vi "Main.vi"() -> ()   [LabVIEW 2015, in "Stock.lvlib"]
doc: "This template is based off of the Queued Message Handler design pattern and the Queued Message Handler project template that ships with LabVIEW.\n\nThe main difference is that the queue is private to this module and communication between modules is performed via Broadcast and Request events.\n\nRequest events are wrapped in public API methods and are handled in the Event Handling Loop (EHL) of this VI. Any module can register for Broadcast events sent by this module. The EHL generates messages based on user interface actions.\n\nThe Message Handling Loop (MHL) processes messages generated by the EHL, or by other messages. The messages are string values, so new messages can be added easily to the Message Cases case structure in the MHL. Each message cluster can also provide an optional value for Message Data, which is a variant that can be converted to whatever message-specific data is required.\n_____\nBased on Delacor QMH Project Template 4.2.1.64."
uses:
  Stock.lvlib
  <vilib>/Delacor/Delacor QMH/Libraries/Module Admin_class/Delacor_lib_QMH_Module Admin.lvclass
  Module Data--cluster.ctl
  Products.ctl
  <vilib>/Delacor/Delacor QMH/Libraries/Message Queue_class/Delacor_lib_QMH_Message Queue.lvclass/Delacor_lib_QMH_Message Queue.ctl
  Stop Argument--cluster.ctl
  <vilib>/Delacor/Delacor QMH/Libraries/Module Admin_class/Delacor_lib_QMH_Module Admin.lvclass/Delacor_lib_QMH_Module Admin.ctl
  In Stock and Price Argument--cluster.ctl
  In Stock and Price (Reply Payload)--cluster.ctl
  Reduce Stock Level Argument--cluster.ctl
  Reduce Stock Level (Reply Payload)--cluster.ctl
  <vilib>/Utility/miscctls.llb/LVPointTypeDef.ctl
  <vilib>/Delacor/Delacor QMH/Libraries/Message Queue_class/Delacor_lib_QMH_Enqueue Message (Single).vi
  <vilib>/Delacor/Delacor QMH/Libraries/Module Admin_class/Delacor_lib_QMH_Get External Launch.vi
  <vilib>/Utility/error.llb/Error Cluster From Error Code.vi
  <vilib>/ErrorRing/Error Ring.xnode
  <vilib>/Delacor/Delacor QMH/Libraries/Message Queue_class/Delacor_lib_QMH_Message Queue.lvclass
panel:
  in  "Subpanel Ref":refnum<vi>
  out "Stock Levels":T1(array[cluster]) {"Price" format="£%.2f"; "Stock Level" scale=0.0..58.0}
  in  "Simulate MHL Error":bool
  in  "Simulate EHL Error":bool
  out "error out":errorcluster
  in  "Module Admin":refnum<class "Delacor_lib_QMH_Module Admin.lvclass">
  out "Status":string
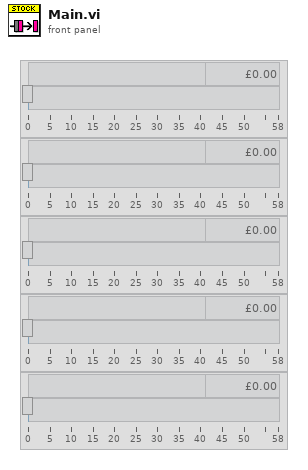
[diagram p1: front panel]
types:
  T1 = cluster{"Name":string, "Price":dbl, "Stock Level":dbl}[]
  T2 = typedef "Stock.lvlib/Request Events--cluster.ctl" = cluster{"Stop Module":refnum<user-event>, "Show Panel":refnum<user-event>, "Hide Panel":refnum<user-event>, "Get Module Execution Status":refnum<user-event>, "Show Diagram":refnum<user-event>, "In Stock and Price":refnum<user-event>, "Reduce Stock Level":refnum<user-event>}
  T3 = typedef "Stock.lvlib/Module Data--cluster.ctl" = cluster{"Status":string, "Stock":T4[], "Stock File Path":path}
  T4 = typedef "Stock.lvlib/Products.ctl" = cluster{"Name":string, "Price (pence/cents)":u32, "Stock Level":u32}
  T5 = enum32{"invalid lock state", "Not Locked", "Locked (No Password)", "Password-protected"}
  T6 = typedef "Stock.lvlib/Stop Argument--cluster.ctl" = cluster{"Origin":string, "Exit via Stop Module Req?":bool, "Wait for Module to stop?":bool}
  T7 = typedef "Stock.lvlib/In Stock and Price Argument--cluster.ctl" = cluster{"Stock Item":u32, "Wait Notifier":refnum<notifier>, "wait for reply":bool}
  T8 = typedef "Stock.lvlib/Reduce Stock Level Argument--cluster.ctl" = cluster{"Product":i32, "Wait Notifier":refnum<notifier>, "wait for reply":bool}
  T9 = typedef "LVPointTypeDef.ctl" = cluster{"Horizontal":i16, "Vertical":i16}
  T10 = typedef "Stock.lvlib/In Stock and Price (Reply Payload)--cluster.ctl" = cluster{"In Stock?":bool, "Price (Pence)":u32, "In Stock and Price_error":errorcluster}
  T11 = typedef "Stock.lvlib/Reduce Stock Level (Reply Payload)--cluster.ctl" = cluster{"Sucessful?":bool, "Reduce Stock Level_error":errorcluster}
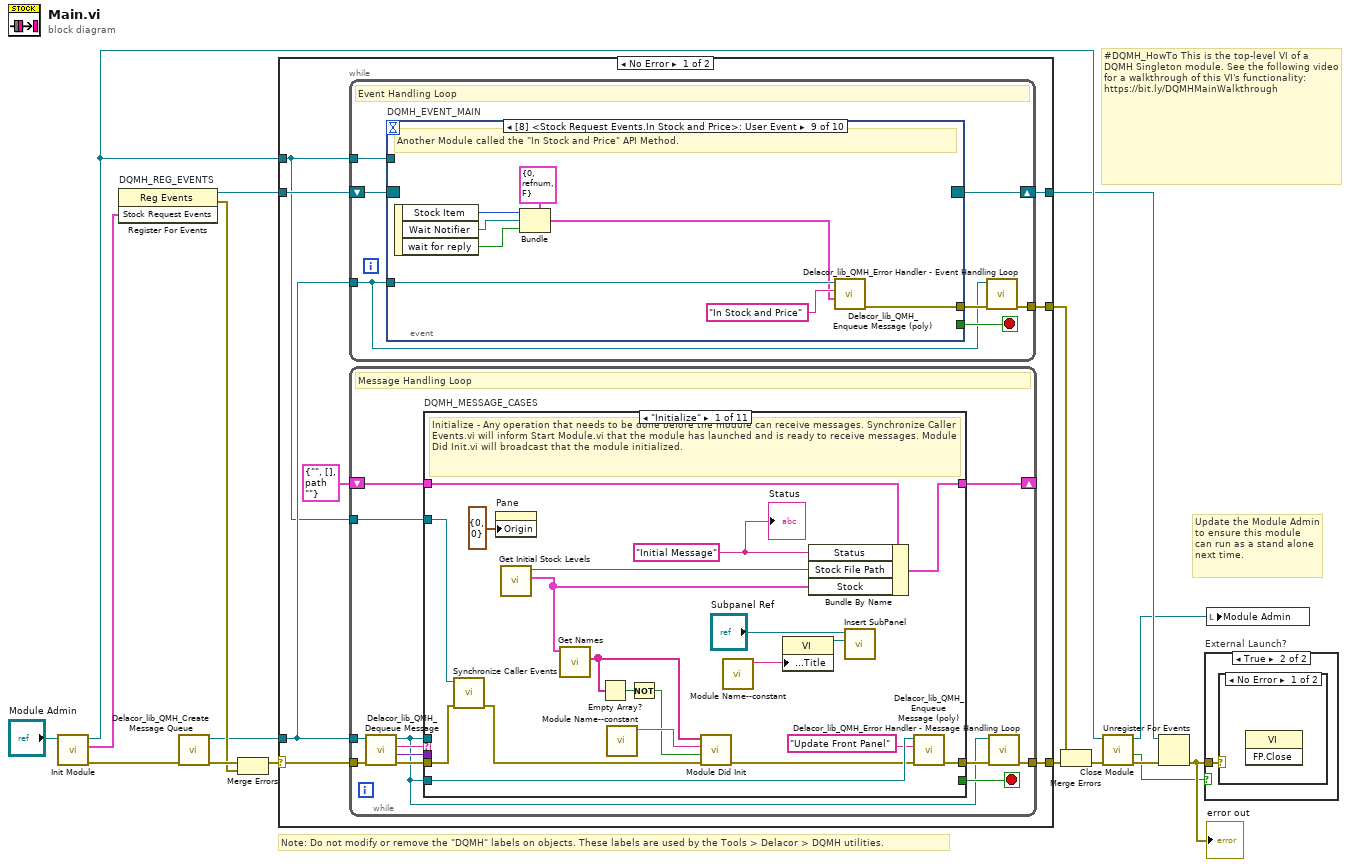
[diagram p0: block diagram]
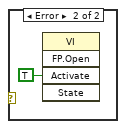
[diagram p3: hidden frame]
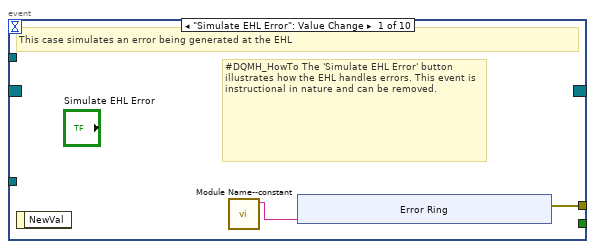
[diagram p4: hidden frame]
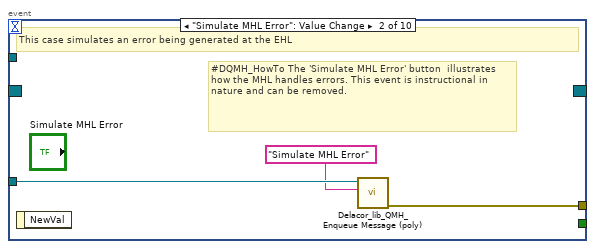
[diagram p5: hidden frame]
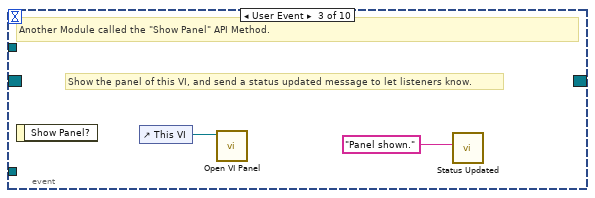
[diagram p6: hidden frame]
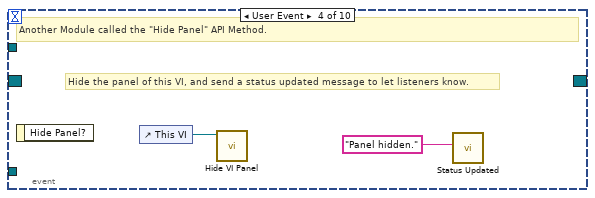
[diagram p7: hidden frame]
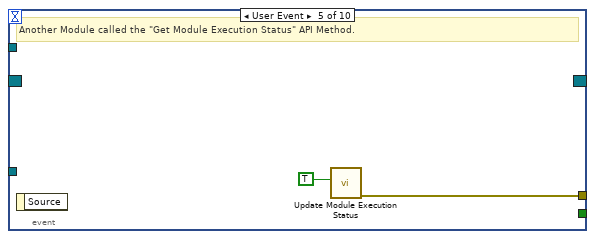
[diagram p8: hidden frame]
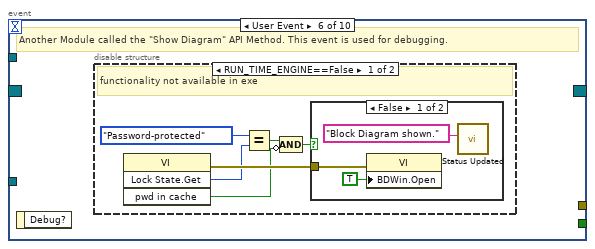
[diagram p9: hidden frame]
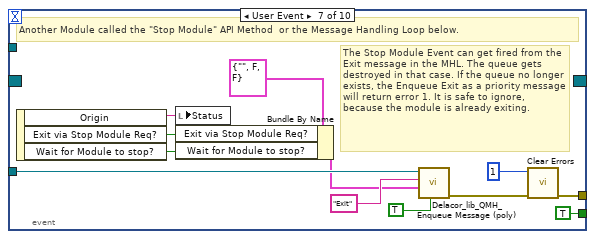
[diagram p12: hidden frame]
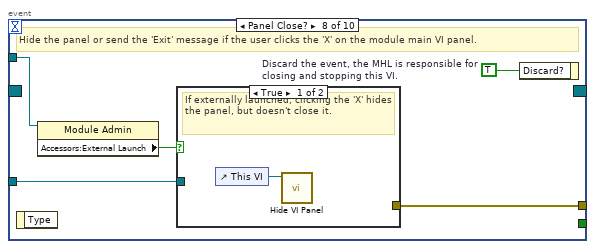
[diagram p13: hidden frame]
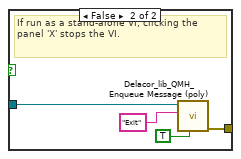
[diagram p14: hidden frame]
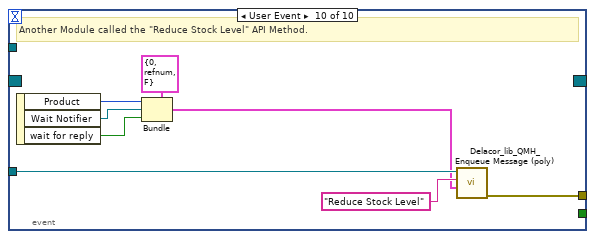
[diagram p15: hidden frame]
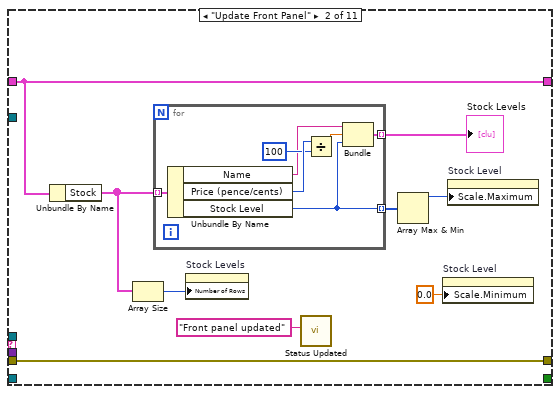
[diagram p16: hidden frame]
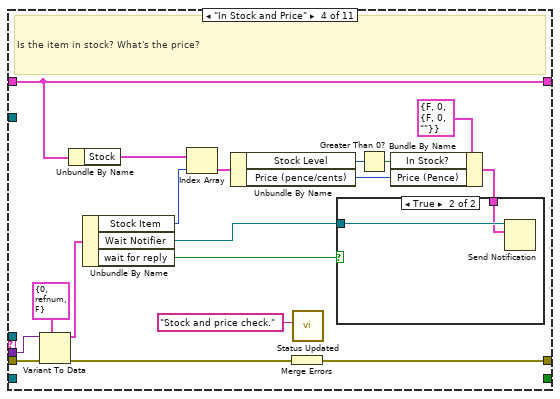
[diagram p18: hidden frame]
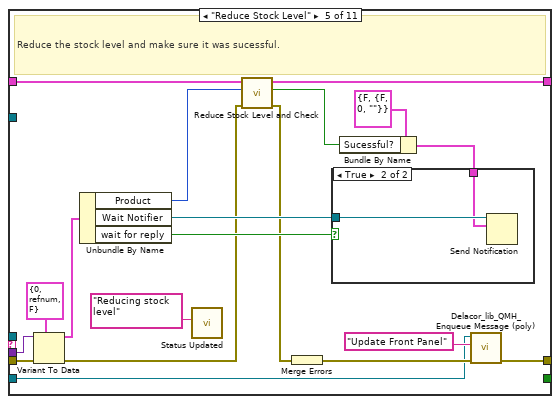
[diagram p20: hidden frame]
diagram:
  # "#DQMH_HowTo This is the top-level VI of a DQMH Singleton module. See the following video for a walkthrough of this VI's functionality: https://bit.ly/DQMHMainWalkthrough"
  # "Note: Do not modify or remove the \"DQMH\" labels on objects. These labels are used by the Tools > Delacor > DQMH utilities."
  # "Update the Module Admin to ensure this module can run as a stand alone next time."
  n1 = call "Init Module.vi"("Singleton Module Admin in"="Module Admin") -> ("error out"=w16:errorcluster, "Stock Request Events"=w5:T2, "Singleton Module Admin out"=w8:refnum<class "Delacor_lib_QMH_Module Admin.lvclass">)  [unwired: 8 in]
  n2 = register-events "DQMH_REG_EVENTS"(w5) -> (reference out=w6:refnum<event-registration>, error out=w9:errorcluster)  [unwired: 2 in]
  n3 = call <vilib>:"Delacor_lib_QMH_Create Message Queue.vi"("error in (no error)"=w16) -> ("error out"=w11:errorcluster, "Message Queue"=w4:refnum<class "Delacor_lib_QMH_Message Queue.lvclass">)  [unwired: 9 in]
  n4 = Merge Errors(w11, w9) -> (w10:errorcluster)
  n5 = case shown="No Error" w10 {
    selector: w10 -> [w23 w258]
    tunnel: [w25 w258] -> w17
    tunnel: [w22 w255] -> w7
    tunnel: w6 -> [w20 w255]
    tunnel: w4 -> [w19 _]
    tunnel: [w24 _] -> w14
    tunnel: w8 -> [w18 w251]
    frame No Error {
      n6 = while {
        tunnel: w19 -> [w26]
        shift-right: [w29] -> w22
        shift-left: w20 -> [w30]
        tunnel: [w31] -> w24
        tunnel: w18 -> [w27]
        stop <- w28 stop-if-true
        # "Event Handling Loop"
        n7 = event "DQMH_EVENT_MAIN" shown="[8] <Stock Request Events.In Stock and Price>: User Event" {
          selector: w30 -> [_ _ _ _ _ _ _ _ _ _]
          dyn-events: [_ _ _ _ _ _ _ _ _ _] -> w29
          timeout: _ -> [_ _ _ _ _ _ _ _ _ _]
          tunnel: [_ _ _ _ _ _ TRUE ("Discard?") _ _ _] -> w28
          tunnel: w26 -> [_ w43 _ _ _ _ w67 w74 w89 w97]
          tunnel: [w34 w44 _ _ w50 _ w70 w76 w82 w90] -> w32
          tunnel: w27 -> [_ _ _ _ _ _ _ w73 _ _]
          event "Simulate EHL Error": Value Change {
            # "#DQMH_HowTo The 'Simulate EHL Error' button  illustrates how the EHL handles errors. This event is instructional in nature and can be removed."
            # "This case simulates an error being generated at the EHL"
            n8 = event-data() -> ()  [unwired: 1 in, 1 out]
            n9 = call "Module Name--constant.vi"() -> ("Module Name"=w33:string)  [unwired: 11 in]
            n10 = xnode "Error Ring"("parameter 0"=w33) -> ("error out"=w34:errorcluster)
          }
          event "Simulate MHL Error": Value Change {
            # "#DQMH_HowTo The 'Simulate MHL Error' button  illustrates how the MHL handles errors. This event is instructional in nature and can be removed."
            # "This case simulates an error being generated at the EHL"
            n11 = event-data() -> ()  [unwired: 1 in, 1 out]
            n12 = call-poly <vilib>:"Delacor_lib_QMH_Enqueue Message (poly).vi"("Message"="Simulate MHL Error", "Message Queue in"=w43) -> ("error out"=w44:errorcluster)  [unwired: 8 in, 1 out]
          }
          event User Event {
            # "Show the panel of this VI, and send a status updated message to let listeners know."
            # "Another Module called the \"Show Panel\" API Method."
            n13 = event-data() -> ()  [unwired: 1 in, 1 out]
            n14 = control-ref of="This VI"() -> (w46:refnum<vi>)
            n15 = call "Open VI Panel.vi"("VI"=w46) -> ()  [unwired: 10 in, 1 out]
            n16 = call "Status Updated.vi"("Status"="Panel shown." ("format string")) -> ()  [unwired: 10 in, 1 out]
          }
          event User Event {
            # "Hide the panel of this VI, and send a status updated message to let listeners know."
            # "Another Module called the \"Hide Panel\" API Method."
            n17 = event-data() -> ()  [unwired: 1 in, 1 out]
            n18 = control-ref of="This VI"() -> (w48:refnum<vi>)
            n19 = call "Hide VI Panel.vi"("VI"=w48) -> ()  [unwired: 10 in, 1 out]
            n20 = call "Status Updated.vi"("Status"="Panel hidden." ("format string")) -> ()  [unwired: 10 in, 1 out]
          }
          event User Event {
            # "Another Module called the \"Get Module Execution Status\" API Method."
            n21 = event-data() -> ()  [unwired: 1 in, 1 out]
            n22 = call "Update Module Execution Status.vi"("Running?"=TRUE) -> ("error out"=w50:errorcluster)  [unwired: 10 in]
          }
          event User Event {
            # "Another Module called the \"Show Diagram\" API Method. This event is used for debugging."
            n23 = event-data() -> ()  [unwired: 1 in, 1 out]
            n24 = disable-structure shown="RUN_TIME_ENGINE==False" {
              frame condition #0 (active) {
                # "functionality not available in exe"
                n25 = invoke class="VI" method="Lock State.Get"() -> (error out=w56:errorcluster, "Get Lock State"=w55:T5, "pwd in cache"=w52:bool)  [unwired: 4 in, 1 out]
                n26 = Equal?(x=T5."Password-protected", y=w55) -> (x = y?=w53:bool)
                n27 = Compound Arithmetic op=AND(w53, invert w52) -> (w51:bool)
                n28 = case shown="False" w51 {
                  tunnel: w56 -> [w59 _]
                  frame False {
                    n29 = property class="VI"(error in=w59, "BDWin.Open"=TRUE ("Block Diagram Window:Open")) -> ()  [unwired: 1 in, 2 out]
                    n30 = call "Status Updated.vi"("Status"="Block Diagram shown." ("format string")) -> ()  [unwired: 10 in, 1 out]
                  }
                  frame True {
                    # "Password-protected VI, and the password is not in the cache. Do not show the diagram."
                  }
                }
              }
              frame condition #1 {
              }
            }
          }
          event User Event {
            # "The Stop Module Event can get fired from the Exit message in the MHL. The queue gets destroyed in that case. If the queue no longer exists, the Enqueue Exit as a priority message will return error 1. It is safe to ignore, because the module is already exiting."
            # "Another Module called the \"Stop Module\" API Method  or the Message Handling Loop below."
            n31 = event-data() -> ("Origin"=w66:string, "Exit via Stop Module Req?"=w62:bool, "Wait for Module to stop?"=w61:bool)  [unwired: 1 in]
            n32 = local write "Status"(w66) -> ()
            n33 = Bundle By Name(cluster=T6 {"Origin"="", "Exit via Stop Module Req?"=FALSE, "Wait for Module to stop?"=FALSE} ("Stop Argument"), "Exit via Stop Module Req?"=w62, "Wait for Module to stop?"=w61) -> (w60:T6)
            n34 = call-poly <vilib>:"Delacor_lib_QMH_Enqueue Message (poly).vi"("Priority Message? (F)"=TRUE, "Message Data"=w60, "Message"="Exit", "Message Queue in"=w67) -> ("error out"=w71:errorcluster)  [unwired: 6 in, 1 out]
            n35 = call <vilib>:"Clear Errors.vi"("error in (no error)"=w71, "specific error code to clear (0: all)"=1) -> ("error out"=w70:errorcluster)  [unwired: 4 in, 1 out]
          }
          event Panel Close? {
            w75 = TRUE  # Discard the event, the MHL is responsible for closing and stopping this VI.
            # "Hide the panel or send the 'Exit' message if the user clicks the 'X' on the module main VI panel."
            n36 = event-data() -> ()  [unwired: 1 in, 1 out]
            n37 = property class="Module Admin"(reference=w73) -> ("Accessors:External Launch"=w72:bool)  [unwired: 1 in, 2 out]
            n38 = case shown="True" w72 {
              tunnel: w74 -> [_ w80]
              tunnel: [_ w81] -> w76
              frame True {
                # "If externally launched, clicking the 'X' hides the panel, but doesn't close it."
                n39 = control-ref of="This VI"() -> (w77:refnum<vi>)
                n40 = call "Hide VI Panel.vi"("VI"=w77) -> ()  [unwired: 10 in, 1 out]
              }
              frame False {
                # "If run as a stand-alone VI, clicking the panel 'X' stops the VI."
                n41 = call-poly <vilib>:"Delacor_lib_QMH_Enqueue Message (poly).vi"("Priority Message? (F)"=TRUE, "Message"="Exit", "Message Queue in"=w80) -> ("error out"=w81:errorcluster)  [unwired: 7 in, 1 out]
              }
            }
            n42 = event-data("Discard?"=w75) -> ()  [unwired: 1 in, 1 out]
          }
          event User Event {
            # "Another Module called the \"In Stock and Price\" API Method."
            n43 = event-data() -> ("Stock Item"=w85:u32, "Wait Notifier"=w84:refnum<notifier>, "wait for reply"=w83:bool)  [unwired: 1 in]
            n44 = Bundle(cluster=T7 {"Stock Item"=0, "Wait Notifier"=refnum, "wait for reply"=FALSE} ("In Stock and Price Argument"), "Stock Item"=w85, "Wait Notifier"=w84, "wait for reply"=w83) -> (w86:T7)
            n45 = call-poly <vilib>:"Delacor_lib_QMH_Enqueue Message (poly).vi"("Message Data"=w86, "Message"="In Stock and Price", "Message Queue in"=w89) -> ("error out"=w82:errorcluster)  [unwired: 7 in, 1 out]
          }
          event User Event {
            # "Another Module called the \"Reduce Stock Level\" API Method."
            n46 = event-data() -> ("Product"=w93:i32, "Wait Notifier"=w92:refnum<notifier>, "wait for reply"=w91:bool)  [unwired: 1 in]
            n47 = Bundle(cluster=T8 {"Product"=0, "Wait Notifier"=refnum, "wait for reply"=FALSE} ("Reduce Stock Level Argument"), "Product"=w93, "Wait Notifier"=w92, "wait for reply"=w91) -> (w94:T8)
            n48 = call-poly <vilib>:"Delacor_lib_QMH_Enqueue Message (poly).vi"("Message Data"=w94, "Message"="Reduce Stock Level", "Message Queue in"=w97) -> ("error out"=w90:errorcluster)  [unwired: 7 in, 1 out]
          }
        }
        n49 = call-dynamic "Delacor_lib_QMH_Error Handler - Event Handling Loop.vi"("error in (no error)"=w32, "Message Queue in"=w26) -> ("dup error in"=w31:errorcluster)  [unwired: 8 in, 1 out]
      }
      n50 = while {
        tunnel: w19 -> [w100]
        shift-right: [w104] -> _
        shift-left: T3 {"Status"="", "Stock"=[], "Stock File Path"=path ""} ("Data Cluster") -> [w105]
        tunnel: w23 -> [w108]
        tunnel: [w106] -> w25
        tunnel: w18 -> [w99]
        stop <- w103 stop-if-true
        # "Message Handling Loop"
        n51 = call-dynamic "Delacor_lib_QMH_Dequeue Message.vi"("error in (no error)"=w108, "Message Queue in"=w100) -> ("error out"=w107:errorcluster, "Message Data"=w101:variant, "Message"=w102:string, "Message Queue out"=w98:refnum<class "Delacor_lib_QMH_Message Queue.lvclass">)  [unwired: 6 in]
        n52 = case "DQMH_MESSAGE_CASES" shown="\"Initialize\"" w102 {
          selector: w102 -> [_ _ _ _ _ _ _ _ _ _ w238]
          tunnel: w98 -> [_ _ _ _ _ _ _ _ w208 w230 _]
          tunnel: w107 -> [w129 w138 w147 w165 w186 w191 w193 w198 w215 w236 w240]
          tunnel: [w118 w138 w147 w156 w170 w190 w193 w197 w211 w233 w241] -> w109
          tunnel: w105 -> [w126 w137 w146 w155 w178 w189 w192 w195 w210 w229 w239]
          tunnel: [w125 w137 w146 w155 w177 w189 w192 w195 w210 w229 w239] -> w104
          tunnel: [_ _ _ _ _ _ _ _ _ w228 _] -> w103
          tunnel: w101 -> [_ _ _ w163 w185 _ _ _ w209 w227 _]
          tunnel: w99 -> [w127 _ _ _ _ _ _ _ w207 w222 _]
          tunnel: w98 -> [w121 _ _ _ w169 _ _ _ _ _ _]
          frame "Initialize" {
            w122 = "Initial Message" ("Initial Message")
            # "Initialize - Any operation that needs to be done before the module can receive messages. Synchronize Caller Events.vi will inform Start Module.vi that the module has launched and is ready to receive messages. Module Did Init.vi will broadcast that the module initialized."
            n53 = call "Synchronize Caller Events.vi"("error in (no error)"=w129, "Singleton Module Admin in"=w127) -> ("error out"=w128:errorcluster)  [unwired: 8 in, 1 out]
            n54 = property on="Pane" class="Pane"("Origin"=T9 {"Horizontal"=0, "Vertical"=0}) -> ()  [unwired: 2 in, 2 out]
            n55 = call "Get Initial Stock Levels.vi"() -> ("Stock"=w114:T4[], "Stock file path"=w113:path)  [unwired: 10 in]
            n56 = call "Get Names.vi"("Stock"=w114) -> ("Product Names"=w110:string[])  [unwired: 10 in]
            n57 = Empty Array?(array=w110) -> (empty?=w112:bool)
            n58 = call "Module Name--constant.vi"() -> ("Module Name"=w124:string)  [unwired: 11 in]
            n59 = Not(x=w112) -> (.not. x?=w111:bool)
            n60 = call "Module Did Init.vi"("error in (no error)"=w128, "Initialized?"=w111, "Origin"=w124, "Product Names"=w110) -> ("error out"=w119:errorcluster)  [unwired: 7 in]
            n61 = call "Module Name--constant.vi"() -> ("Module Name"=w117:string)  [unwired: 11 in]
            n62 = property class="VI"("Front Panel.Title"=w117) -> (reference out=w115:refnum<vi>)  [unwired: 2 in, 1 out]
            n63 = Bundle By Name(cluster=w126, "Status"=w122, "Stock File Path"=w113, "Stock"=w114) -> (w125:T3)
            n64 = call "Insert SubPanel.vi"("VI Ref"=w115, "Subpanel Ref"="Subpanel Ref") -> ()  [unwired: 9 in, 1 out]
            n65 = call-poly <vilib>:"Delacor_lib_QMH_Enqueue Message (poly).vi"("error in (no error)"=w119, "Message"="Update Front Panel" ("Initial Message"), "Message Queue in"=w121) -> ("error out"=w118:errorcluster)  [unwired: 7 in, 1 out]
            "Status" <- w122
          }
          frame "Update Front Panel" {
            n66 = Unbundle By Name(w137) -> ("Stock"=w133:T4[])
            n67 = Array Size(array=w133) -> (size(s)=w132:i32)
            n68 = for {
              tunnel: w133 -> [w145] mode=indexing
              tunnel: [w142] -> w135 mode=indexing
              tunnel: [w139] -> w136 mode=indexing
              n69 = Unbundle By Name(w145) -> ("Name"=w140:string, "Price (pence/cents)"=w144:u32, "Stock Level"=w142:u32)
              n70 = Divide(x=w144, y=u32 100) -> (x/y=w141:dbl)
              n71 = Bundle("Name"=w140, w141, "Stock Level"=w142) -> (w139:cluster{"Name":string, dbl, "Stock Level":u32})  [unwired: 1 in]
            }
            "Stock Levels" <- w136
            n72 = property on="Stock Levels" class="Arr (strict)"("Number of Rows"=w132) -> ()  [unwired: 2 in, 2 out]
            n73 = call "Status Updated.vi"("Status"="Front panel updated") -> ()  [unwired: 10 in, 1 out]
            n74 = Array Max & Min(array=w135) -> (max value=w134:u32)  [unwired: 3 out]
            n75 = property on="Stock Level" class="Slide (strict)"("Scale.Minimum"=0.0 ("Scale.Range:Minimum")) -> ()  [unwired: 2 in, 2 out]
            n76 = property on="Stock Level" class="Slide (strict)"("Scale.Maximum"=w134) -> ()  [unwired: 2 in, 2 out]
          }
          frame "--- Module Specific ---" {
            # "Separator -- The following cases handle messages specific to this Module."
          }
          frame "In Stock and Price" {
            # "Is the item in stock? What's the price?"
            n77 = Variant To Data(error in=w165, type=T7 {"Stock Item"=0, "Wait Notifier"=refnum, "wait for reply"=FALSE} ("In Stock and Price Argument"), Variant=w163) -> (data=w161:T7, error out=w164:errorcluster)
            n78 = Unbundle By Name(w155) -> ("Stock"=w154:T4[])
            n79 = Unbundle By Name(w161) -> ("Stock Item"=w153:u32, "Wait Notifier"=w160:refnum<notifier>, "wait for reply"=w159:bool)
            n80 = Index Array(array=w154, index=w153) -> (element=w152:T4)
            n81 = Unbundle By Name(w152) -> ("Stock Level"=w150:u32, "Price (pence/cents)"=w151:u32)
            n82 = Merge Errors(w164) -> (w156:errorcluster)
            n83 = call "Status Updated.vi"("Status"="Stock and price check.") -> ()  [unwired: 10 in, 1 out]
            n84 = Greater Than 0?(x=w150) -> (x > 0?=w149:bool)
            n85 = Bundle By Name(cluster=T10 {"In Stock?"=FALSE, "Price (Pence)"=0, "In Stock and Price_error"={"status"=FALSE, "code"=0, "source"=""}} ("In Stock and Price (Reply Payload)"), "In Stock?"=w149, "Price (Pence)"=w151) -> (w158:T10)
            n86 = case shown="True" w159 {
              tunnel: w160 -> [_ w167]
              tunnel: w158 -> [_ w166]
              frame False {
              }
              frame True {
                n87 = Send Notification(notification=w166, notifier=w167) -> ()  [unwired: 1 in, 2 out]
              }
            }
          }
          frame "Reduce Stock Level" {
            # "Reduce the stock level and make sure it was sucessful."
            n88 = Variant To Data(error in=w186, type=T8 {"Product"=0, "Wait Notifier"=refnum, "wait for reply"=FALSE} ("Reduce Stock Level Argument"), Variant=w185) -> (data=w183:T8, error out=w174:errorcluster)
            n89 = Unbundle By Name(w183) -> ("Product"=w176:i32, "Wait Notifier"=w182:refnum<notifier>, "wait for reply"=w181:bool)
            n90 = call "Status Updated.vi"("Status"="Reducing stock level") -> ()  [unwired: 10 in, 1 out]
            n91 = call "Reduce Stock Level and Check.vi"("error in (no error)"=w174, "Product Index"=w176, "Data Cluster"=w178) -> ("error out"=w173:errorcluster, "Sucessful"=w175:bool, "Data Cluster Out"=w177:T3)  [unwired: 6 in]
            n92 = Merge Errors(w173) -> (w171:errorcluster)
            n93 = Bundle By Name(cluster=T11 {"Sucessful?"=FALSE, "Reduce Stock Level_error"={"status"=FALSE, "code"=0, "source"=""}} ("Reduce Stock Level (Reply Payload)"), "Sucessful?"=w175) -> (w180:T11)
            n94 = case shown="True" w181 {
              tunnel: w182 -> [_ w188]
              tunnel: w180 -> [_ w187]
              frame False {
              }
              frame True {
                n95 = Send Notification(notification=w187, notifier=w188) -> ()  [unwired: 1 in, 2 out]
              }
            }
            n96 = call-poly <vilib>:"Delacor_lib_QMH_Enqueue Message (poly).vi"("error in (no error)"=w171, "Message"="Update Front Panel" ("Initial Message"), "Message Queue in"=w169) -> ("error out"=w170:errorcluster)  [unwired: 7 in, 1 out]
          }
          frame "---Copy This Frame---" {
            # "Duplicate this frame when creating new messages.  Change this comment in the duplicated frame to describe this message."
            n97 = Merge Errors(w191) -> (w190:errorcluster)
          }
          frame "--- Exit and Error Handling---" {
            # "Separator - The following cases handle errors and exit messages."
          }
          frame "Simulate MHL Error" {
            # "#DQMH_HowTo The 'Simulate MHL Error' button  illustrates how the MHL handles errors. This event is instructional in nature and can be removed."
            # "Simulate an error occurring at the MHL"
            n98 = call "Module Name--constant.vi"() -> ("Module Name"=w194:string)  [unwired: 11 in]
            n99 = xnode "Error Ring"("parameter 0"=w194) -> ("error out"=w196:errorcluster)
            n100 = Merge Errors(w198, w196) -> (w197:errorcluster)
          }
          frame "Error" {
            # "#CodeRecommended - If you ever change the name of this \"Error\" message, you'll need to update the name in the Check Loop Error.vi as well."
            # "#CodeRecommended - If the module is running in standalone mode (External Launch = FALSE), this code will pop up an error dialog and call the 'Exit' message if an error occurs. Add more fine-grained error handling here."
            # "Error - Check the error message data and respond accordingly. This message is sent by the \"Error Handler\" VIs at the end of each loop in this application."
            n101 = property class="Module Admin"(reference=w207) -> ("Accessors:External Launch"=w206:bool)  [unwired: 1 in, 2 out]
            n102 = Variant To Data(error in=w215, type=errorcluster {"status"=FALSE, "code"=0, "source"=""} ("error constant"), Variant=w209) -> (data=w216:errorcluster, error out=w213:errorcluster)
            n103 = call "Error Reported.vi"("Error"=w216) -> ()  [unwired: 10 in, 1 out]
            n104 = case shown="True" w206 {
              tunnel: [w221 _] -> w212
              tunnel: w208 -> [w219 _]
              tunnel: w216 -> [w220 _]
              frame False {
                # "If the module is running standalone, then pop up an error dialog and call the \"Exit\" message."
                n105 = call <vilib>:"Simple Error Handler.vi"("error in (no error)"=w220) -> ()  [unwired: 4 in, 5 out]
                n106 = call-poly <vilib>:"Delacor_lib_QMH_Enqueue Message (poly).vi"("Priority Message? (F)"=TRUE, "Message"="Exit", "Message Queue in"=w219) -> ("error out"=w221:errorcluster)  [unwired: 7 in, 1 out]
              }
              frame True {
                # "If the module was launched externally, calling the Error Reported broadcast VI is the only action performed by the \"Error\" message. The module's caller can then process the error appropriately."
              }
            }
            n107 = Merge Errors(w213, w212) -> (w211:errorcluster)
            n108 = local write "error out"(w211) -> ()
          }
          frame "Exit" {
            w226 = 91  # 91: not all Exit messages will have an argument
            w228 = TRUE  # Stop the VI
            # "Release the message queue reference"
            # "#CodeNeeded - Add any required cleanup code here"
            # "Exit - Exit the application."
            n109 = Variant To Data(error in=w236, type=T6 {"Origin"="", "Exit via Stop Module Req?"=FALSE, "Wait for Module to stop?"=FALSE} ("Stop Argument"), Variant=w227) -> (data=w224:T6, error out=w232:errorcluster)
            n110 = call <vilib>:"Clear Errors.vi"("error in (no error)"=w232, "specific error code to clear (0: all)"=w226) -> ("error out"=w235:errorcluster)  [unwired: 4 in, 1 out]
            n111 = control-ref of="This VI"() -> (w223:refnum<vi>)
            n112 = call-dynamic "Delacor_lib_QMH_Release Message Queue.vi"("error in (no error)"=w235, "Message Queue"=w230) -> ("error out"=w234:errorcluster)  [unwired: 9 in]
            n113 = call "Handle Exit.vi"("Stop Argument"=w224, "Admin in"=w222, "VI reference"=w223) -> ("error out"=w231:errorcluster)  [unwired: 7 in, 1 out]
            n114 = Merge Errors(w234, w231) -> (w233:errorcluster)
          }
          frame Default {
            # "'Default' case only runs if there is a message that isn't defined in any of the other cases.  Output a programming error."
            n115 = call "Module Name--constant.vi"() -> ("Module Name"=w237:string)  [unwired: 11 in]
            n116 = xnode "Error Ring"("parameter 0"=w238, "parameter 1"=w237) -> ("error out"=w242:errorcluster)
            n117 = Merge Errors(w240, w242) -> (w241:errorcluster)
          }
        }
        n118 = call-dynamic "Delacor_lib_QMH_Error Handler - Message Handling Loop.vi"("error in (no error)"=w109, "Message Queue in"=w98) -> ("dup error in"=w106:errorcluster)  [unwired: 8 in, 1 out]
      }
    }
    frame Error {
      # "Synchronize Caller Events.vi will inform Start Module.vi that the module has launched and will let the code calling Start Module.vi register for broadcasts and would permit the caller receive the broadcast that an error occurred at launch time."
      n119 = call "Synchronize Caller Events.vi"("Singleton Module Admin in"=w251) -> ("error out"=w256:errorcluster)  [unwired: 9 in, 1 out]
      n120 = call "Module Name--constant.vi"() -> ("Module Name"=w254:string)  [unwired: 11 in]
      n121 = Format Into String(format string="An error occurred during initialization. %s is no longer running.", w254) -> (resulting string=w252:string)  [unwired: 2 in, 1 out]
      n122 = Merge Errors(w258, w256) -> (w257:errorcluster)
      n123 = call "Error Reported.vi"("Additional Information"=w252, "Error"=w257) -> ()  [unwired: 9 in, 1 out]
    }
  }
  n124 = Merge Errors(w14, w17) -> (w13:errorcluster)
  n125 = call "Close Module.vi"("error in (no error)"=w13, "Module Admin in"=w8) -> ("error out"=w15:errorcluster, "External Launch"=w1:bool, "Module Admin out"=w2:refnum<class "Delacor_lib_QMH_Module Admin.lvclass">)  [unwired: 7 in]
  n126 = Unregister For Events(event registration refnum=w7, error in=w15) -> (error out=w12:errorcluster)
  "error out" <- w12
  n127 = case "External Launch?" shown="True" w1 {
    tunnel: w12 -> [_ w259]
    frame False {
    }
    frame True {
      n128 = case shown="No Error" w259 {
        frame No Error {
          n129 = invoke class="VI" method="FP.Close"() -> ()  [unwired: 3 in, 3 out]
        }
        frame Error {
          n130 = invoke class="VI" method="FP.Open"("Activate"=TRUE ("Activate?")) -> ()  [unwired: 4 in, 5 out]
        }
      }
    }
  }
  n131 = local write "Module Admin"(w2) -> ()
